vi "DTbl Compress Digital.vi"(7 "force compression?":bool, 8 "error in (no error)":errorcluster, 11 "uncompressed digital data":digitaldata) -> (0 "error out":errorcluster, 3 "compressed digital data":digitaldata)   [LabVIEW 2020]
doc: "Compresses the digital signals in the digital input and returns the result in the digital output. Wire data to the <B>uncompressed digital waveform</B> input to determine the polymorphic instance to use or manually select the instance."
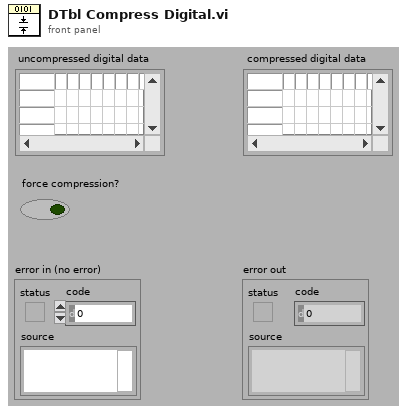
[diagram p1: front panel]
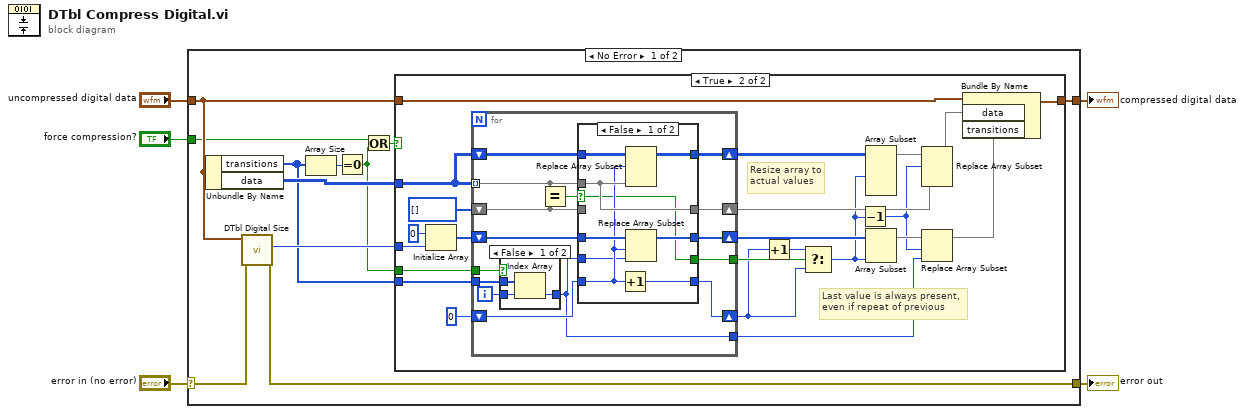
[diagram p0: block diagram]
diagram:
  n1 = case shown="No Error" "error in (no error)" {
    selector: "error in (no error)" -> [w10 w75]
    tunnel: [w16 w74] -> w5
    tunnel: "uncompressed digital data" -> [w13 w74]
    tunnel: [w11 w75] -> w3
    tunnel: "force compression?" -> [w8 _]
    frame No Error {
      n2 = Unbundle By Name(w13) -> ("transitions"=w6:u32[], "data"=w12:u8[][])
      n3 = call "DTbl Digital Size.vi"("error in (no error)"=w10, "digital data in"=w13) -> ("error out"=w11:errorcluster, "number of samples"=w14:i32)  [unwired: 6 in, 2 out]
      n4 = Array Size(array=w6) -> (size(s)=w15:i32)
      n5 = Equal To 0?(x=w15) -> (x = 0?=w7:bool)
      n6 = Or(x=w8, y=w7) -> (x .or. y?=w9:bool)
      n7 = case shown="True" w9 {
        tunnel: [w17 w22] -> w16
        tunnel: w12 -> [_ w39]
        tunnel: w14 -> [_ w30]
        tunnel: w13 -> [w17 w24]
        tunnel: w7 -> [_ w19]
        tunnel: w6 -> [_ w18]
        frame False {
          # "Already Compressed"
        }
        frame True {
          # "Last value is always present,\neven if repeat of previous"
          # "Resize array to\nactual values"
          n8 = Initialize Array(u32 0, w30) -> (w37:u32[])
          n9 = for {
            shift-right: [w54] -> w36
            shift-left: w39 -> [w55]
            shift-right: [w49] -> w20
            shift-left: 0 -> [w50]
            tunnel: w39 -> [w52] mode=indexing
            shift-right: [w53] -> w34
            shift-left: i8[] [] ("Data") -> [w51]
            shift-right: [w47] -> w33
            shift-left: w37 -> [w48]
            tunnel: [w41] -> w31
            tunnel: [w46] -> w25
            tunnel: w19 -> [w44]
            tunnel: w18 -> [w43]
            i -> [w42]
            n10 = case shown="False" w44 {
              tunnel: [w58 w59] -> w41
              tunnel: w42 -> [w57 w59]
              tunnel: w43 -> [w56 _]
              frame False {
                n11 = Index Array(array=w56, index=w57) -> (element=w58:u32)
              }
              frame True {
              }
            }
            n12 = Equal?(x=w52, y=w51) -> (x = y?=w45:bool)
            n13 = case shown="False" w45 {
              selector: w45 -> [w60 w69]
              tunnel: w55 -> [w68 w73]
              tunnel: [w67 w73] -> w54
              tunnel: [w66 w72] -> w53
              tunnel: w52 -> [w66 _]
              tunnel: w51 -> [_ w72]
              tunnel: [w65 w71] -> w49
              tunnel: w50 -> [w63 w71]
              tunnel: w48 -> [w64 w70]
              tunnel: [w62 w70] -> w47
              tunnel: w41 -> [w61 _]
              tunnel: [w60 w69] -> w46
              frame False {
                n14 = Increment(x=w63) -> (x+1=w65:i32)
                n15 = Replace Array Subset(array=w68, new element=w66, index (row)=w63) -> (w67:u8[][])  [unwired: 1 in]
                n16 = Replace Array Subset(array=w64, new element=w61, index=w63) -> (w62:u32[])
              }
              frame True {
                # "Same value as\nprevious - ignore"
              }
            }
          }
          n17 = Increment(x=w20) -> (x+1=w27:i32)
          n18 = Select(t=w27, s=w25, f=w20) -> (s? t:f=w26:i32)
          n19 = Decrement(x=w26) -> (x-1=w28:i32)
          n20 = Array Subset(array=w36, length (row)=w26) -> (w35:u8[][])  [unwired: 3 in]
          n21 = Array Subset(array=w33, length=w26) -> (w32:u32[])  [unwired: 1 in]
          n22 = Replace Array Subset(array=w35, new element=w34, index (row)=w28) -> (w21:u8[][])  [unwired: 1 in]
          n23 = Replace Array Subset(array=w32, new element=w31, index=w28) -> (w23:u32[])
          n24 = Bundle By Name(cluster=w24, "data"=w21, "transitions"=w23) -> (w22:digitaldata)
        }
      }
    }
    frame Error {
    }
  }
  "compressed digital data" <- w5
  "error out" <- w3
